vi "Initialize Hardware References.vi"(8 "error in (no error)":cluster{"状态":bool, "代码":i32, "源":string} caption="错误输入（无错误）", 11 "硬件资源输入":T1) -> (0 "error out":cluster{"状态":bool, "代码":i32, "源":string} caption="错误输出", 3 "硬件资源输出":T1)   [LabVIEW 2014, in "Acquisition.lvlib"]
doc: "初始化硬件引用。"
uses:
  Acquisition.lvlib
  Hardware Configuration.ctl
  Signal Type.ctl
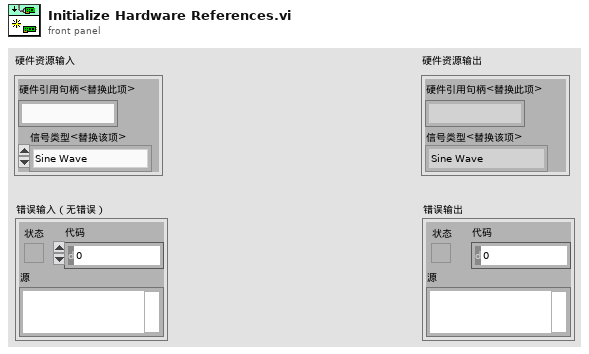
[diagram p1: front panel]
types:
  T1 = typedef "Acquisition.lvlib/Hardware Configuration.ctl" = cluster{"硬件引用句柄<替换此项>":string, "信号类型<替换该项>":T2}
  T2 = typedef "Acquisition.lvlib/Signal Type.ctl" = enum16{"Sine Wave", "Square with Noise"}
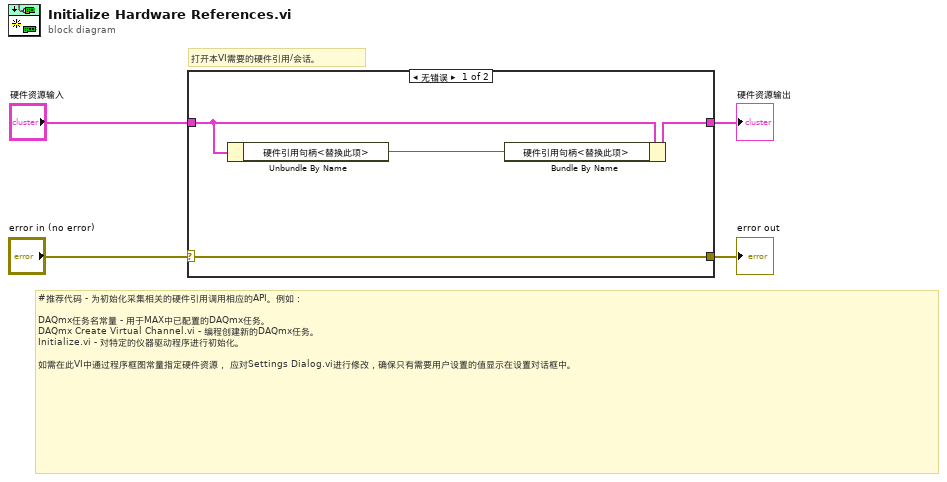
[diagram p0: block diagram]
diagram:
  # "打开本VI需要的硬件引用/会话。"
  # "#推荐代码 - 为初始化采集相关的硬件引用调用相应的API。例如：\n\nDAQmx任务名常量 - 用于MAX中已配置的DAQmx任务。\nDAQmx Create Virtual Channel.vi - 编程创建新的DAQmx任务。\nInitialize.vi - 对特定的仪器驱动程序进行初始化。\n\n如需在此VI中通过程序框图常量指定硬件资源， 应对Settings Dialog.vi进行修改，确保只有需要用户设置的值显示在设置对话框中。"
  n1 = case shown="无错误" "error in (no error)" {
    selector: "error in (no error)" -> [w7 w9]
    tunnel: [w7 w9] -> w3
    tunnel: "硬件资源输入" -> [w6 w10]
    tunnel: [w8 w10] -> w1
    frame No Error {
      n2 = Unbundle By Name(w6) -> ("硬件引用句柄<替换此项>"=w5:string)
      n3 = Bundle By Name(cluster=w6, "硬件引用句柄<替换此项>"=w5) -> (w8:T1)
    }
    frame Error {
    }
  }
  "硬件资源输出" <- w1
  "error out" <- w3
